vi "QueryLaserConfigLCDC501.vi"(8 "error in (no error)":errorcluster, 11 "VISA resource name":refnum<visa-resource-name>) -> (0 "error out":errorcluster, 2 "LASER CONFIGURATION":T1={"LD Range"=1, "Laser Control Mode"=0, "Laser Mod On/OFF"=1, "Laser Mod BW"=1} {"Laser Mod BW" items=["Low", "High"]; "Laser Mod On/OFF" items=["OFF", "ON"]; "Laser Control Mode" items=["CC", "CP"]; "LD Range" items=["250mA", "500mA"]}, 3 "VISA resource name out":refnum<visa-resource-name>)   [LabVIEW 2021]
panel:
  # "LD Currernt Range"
  # "Laser Control Mode"
  # "Laser Mod On/OFF"
  # "Laser Mod BW"
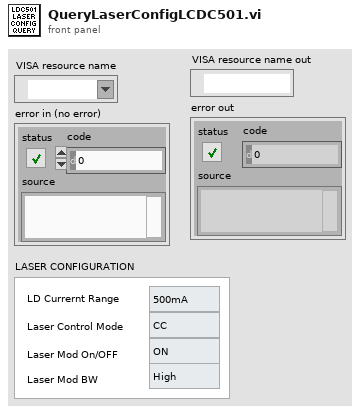
[diagram p1: front panel]
types:
  T1 = cluster{"LD Range":u16, "Laser Control Mode":u16, "Laser Mod On/OFF":u16, "Laser Mod BW":u16}
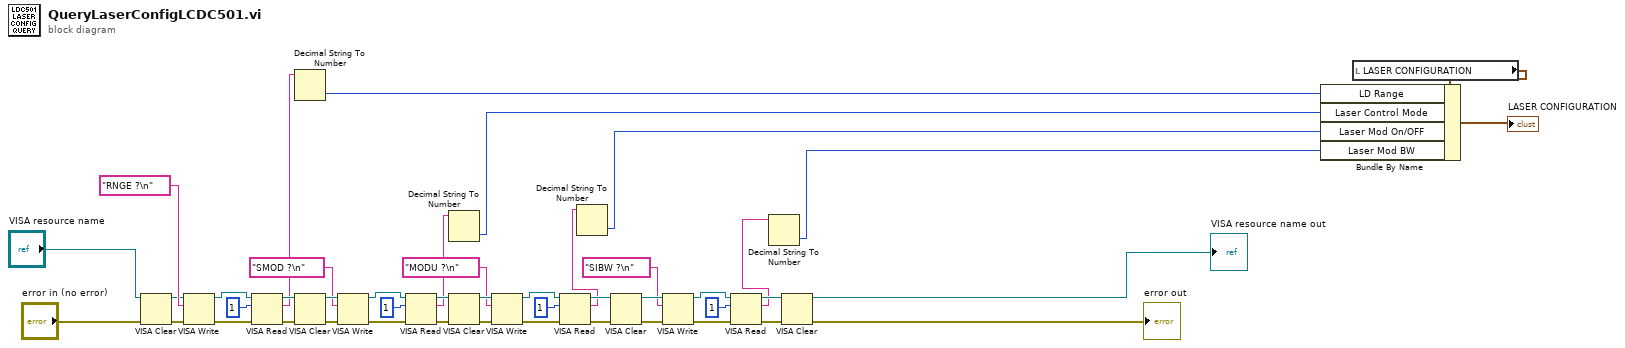
[diagram p0: block diagram]
diagram:
  n1 = VISA Clear(VISA resource name="VISA resource name", error in (no error)="error in (no error)") -> (VISA resource name out=w41:refnum<visa-resource-name>, error out=w42:errorcluster)
  n2 = VISA Write(VISA resource name=w41, write buffer="RNGE ?\n", error in (no error)=w42) -> (VISA resource name out=w45:refnum<visa-resource-name>, error out=w44:errorcluster)  [unwired: 1 out]
  n3 = VISA Read(VISA resource name=w45, byte count=u32 1, error in (no error)=w44) -> (VISA resource name out=w22:refnum<visa-resource-name>, read buffer=w12:string, error out=w21:errorcluster)  [unwired: 1 out]
  n4 = Decimal String To Number(string=w12) -> (number=w10:i32)  [unwired: 2 in, 1 out]
  n5 = VISA Clear(VISA resource name=w22, error in (no error)=w21) -> (VISA resource name out=w37:refnum<visa-resource-name>, error out=w38:errorcluster)
  n6 = VISA Write(VISA resource name=w37, write buffer="SMOD ?\n", error in (no error)=w38) -> (VISA resource name out=w40:refnum<visa-resource-name>, error out=w39:errorcluster)  [unwired: 1 out]
  n7 = VISA Read(VISA resource name=w40, byte count=u32 1, error in (no error)=w39) -> (VISA resource name out=w33:refnum<visa-resource-name>, read buffer=w11:string, error out=w31:errorcluster)  [unwired: 1 out]
  n8 = Decimal String To Number(string=w11) -> (number=w9:i32)  [unwired: 2 in, 1 out]
  n9 = VISA Clear(VISA resource name=w33, error in (no error)=w31) -> (VISA resource name out=w32:refnum<visa-resource-name>, error out=w34:errorcluster)
  n10 = VISA Write(VISA resource name=w32, write buffer="MODU ?\n", error in (no error)=w34) -> (VISA resource name out=w35:refnum<visa-resource-name>, error out=w36:errorcluster)  [unwired: 1 out]
  n11 = VISA Read(VISA resource name=w35, byte count=u32 1, error in (no error)=w36) -> (VISA resource name out=w26:refnum<visa-resource-name>, read buffer=w7:string, error out=w25:errorcluster)  [unwired: 1 out]
  n12 = Decimal String To Number(string=w7) -> (number=w6:i32)  [unwired: 2 in, 1 out]
  n13 = VISA Clear(VISA resource name=w26, error in (no error)=w25) -> (VISA resource name out=w27:refnum<visa-resource-name>, error out=w28:errorcluster)
  n14 = VISA Write(VISA resource name=w27, write buffer="SIBW ?\n", error in (no error)=w28) -> (VISA resource name out=w29:refnum<visa-resource-name>, error out=w30:errorcluster)  [unwired: 1 out]
  n15 = VISA Read(VISA resource name=w29, byte count=u32 1, error in (no error)=w30) -> (VISA resource name out=w24:refnum<visa-resource-name>, read buffer=w5:string, error out=w23:errorcluster)  [unwired: 1 out]
  n16 = Decimal String To Number(string=w5) -> (number=w4:i32)  [unwired: 2 in, 1 out]
  n17 = VISA Clear(VISA resource name=w24, error in (no error)=w23) -> (VISA resource name out=→"VISA resource name out":refnum<visa-resource-name>, error out=→"error out":errorcluster)
  n18 = local read "LASER CONFIGURATION"() -> (w8:T1)
  n19 = Bundle By Name(cluster=w8, "LD Range"=w10, "Laser Control Mode"=w9, "Laser Mod On/OFF"=w6, "Laser Mod BW"=w4) -> (→"LASER CONFIGURATION":T1)
